vi "Select_Ref.vi"(4 "Nazwa pliku":refnum<vi>, 6 "Path in":refnum<vi>, 8 "error in (no error)":errorcluster, 11 "NewVal":string) -> (0 "error out":errorcluster)   [LabVIEW 2021]
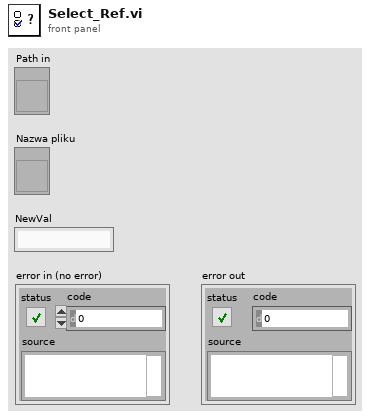
[diagram p1: front panel]
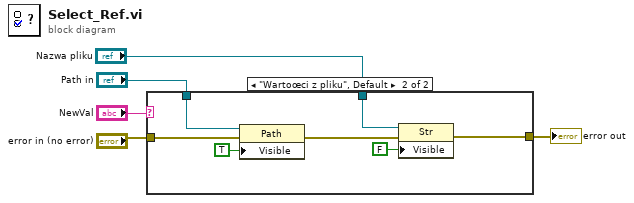
[diagram p0: block diagram]
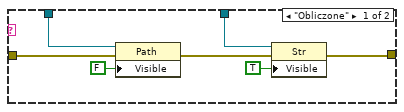
[diagram p2: hidden frame]
diagram:
  n1 = case shown="\"Wartoœci z pliku\", Default" "NewVal" {
    tunnel: "Path in" -> [w6 w18]
    tunnel: "Nazwa pliku" -> [w7 w14]
    tunnel: "error in (no error)" -> [w10 w17]
    tunnel: [w8 w13] -> w5
    frame "Obliczone" {
      n2 = property class="Path"(reference=w6, error in=w10, "Visible"=FALSE) -> (error out=w9:errorcluster)  [unwired: 1 out]
      n3 = property class="Str"(reference=w7, error in=w9, "Visible"=TRUE) -> (error out=w8:errorcluster)  [unwired: 1 out]
    }
    frame "Wartoœci z pliku", Default {
      n4 = property class="Path"(reference=w18, error in=w17, "Visible"=TRUE) -> (error out=w15:errorcluster)  [unwired: 1 out]
      n5 = property class="Str"(reference=w14, error in=w15, "Visible"=FALSE) -> (error out=w13:errorcluster)  [unwired: 1 out]
    }
  }
  "error out" <- w5
